vi "movedelaySD.vi"(0 "Delay, mm":dbl) -> (1 "Real delay time, ps":dbl=3790.0, 2 "Pos, mm":dbl)   [LabVIEW 2015]
uses:
  globalVarSD.vi
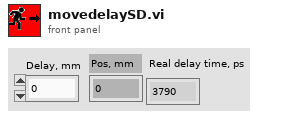
[diagram p1: front panel]
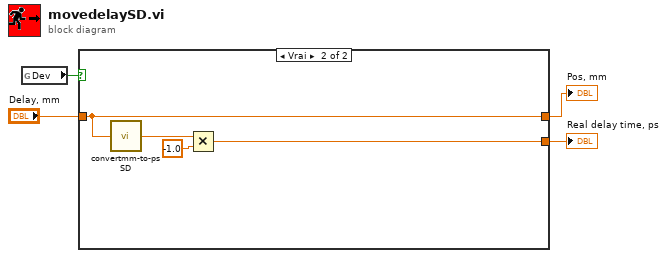
[diagram p0: block diagram]
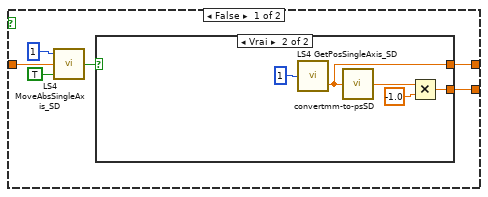
[diagram p2: hidden frame]
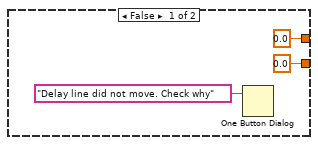
[diagram p3: hidden frame]
diagram:
  n1 = global read "globalVarSD.vi" "Dev"() -> (w3:bool)
  n2 = case shown="Vrai" w3 {
    tunnel: "Delay, mm" -> [w10 w20]
    tunnel: [w6 w19] -> w2
    tunnel: [w5 w20] -> w1
    frame False {
      n3 = call "LS4 MoveAbsSingleAxis_SD.vi"("Wait"=TRUE, "Value"=w10, "Axis"=1) -> ("Command executed"=w9:bool)
      n4 = case shown="Vrai" w9 {
        tunnel: [0.0 w15] -> w6
        tunnel: [0.0 ("Pos") w14] -> w5
        frame False {
          n5 = One Button Dialog(message="Delay line did not move. Check why") -> ()  [unwired: 1 in, 1 out]
        }
        frame True {
          n6 = call "LS4 GetPosSingleAxis_SD.vi"("Axis"=1) -> ("Pos"=w14:dbl)  [unwired: 1 out]
          n7 = call "convertmm-to-psSD.vi"("mm"=w14) -> ("ps"=w17:dbl)
          n8 = Multiply(x=w17, y=-1.0) -> (x*y=w15:dbl)
        }
      }
    }
    frame True {
      n9 = call "convertmm-to-psSD.vi"("mm"=w20) -> ("ps"=w22:dbl)
      n10 = Multiply(x=w22, y=-1.0) -> (x*y=w19:dbl)
    }
  }
  "Real delay time, ps" <- w2
  "Pos, mm" <- w1
